vi "Simulation - Tank Level.vi"() -> ()   [LabVIEW 2023]
doc: "This example demonstrates a process simulation for a tank level. The process has added noise, valve deadband, lag, and deadtime. A level controller adjusts the inflow to a tank. An on/off valve serves as a drain that you can click on to operate. This s-valve represents a change in the process loading. You also can switch this VI from automatic control to manual control."
uses:
  <vilib>/addons/control/pid/pid.llb/PID Advanced (DBL).vi
  <vilib>/addons/control/pid/NI_PID_pid.lvlib
panel:
  in  "Tab Control":enum32{"Introduction", "Operation"}(tab)
  out "Flow sensor":bool
  in  "HV-101":bool
  out "tank level":dbl(slide) scale=0.0..100.0 scale format="%#.2g"
  out "Valve":bool
  in  "LCV-101":dbl(knob) scale=0.0..100.0
  in  "Auto":bool=TRUE
  out "Process Chart":T1(graph)={"initial PV"=18.934717983735947, "SP(%)"=34.59119496855346, "output"=100.0}
  in  "Setpoint":dbl(slide)=50.0 scale=0.0..100.0
  in  "PID parameters (LIC 101)":T2={"Kc"=10.0, "Ti (min)"=0.05, "Td (min)"=0.0} {"Td (min)" format="%#.6f"; "Ti (min)" format="%#.4f"; "Kc" format="%#.4f"}
  in  "Stop":bool
  # "Tank Level Control"
  # "Overview: This example demonstrates a process simulation for a tank level.  The process has added noise, valve deadband, lag, and deadtime.  A level controller adjusts the inflow to a tank.  An on/off valve serves as a drain that you can click on to operate.  This s-valve represents a change in the process loading.  You also can switch this VI from automatic control to manual control.\nInstructions:\n1. Run the VI.\n2. Verify the PID controller in closed-loop to track the setpoint.\n3. Change the setpoint to another value and verify the controller tracking the new setpoint.\n4. Apply a disturbance to the system by switching the valve HV 102 (click on the valve symbol). You will see the controller recovering fro the change.\n5. Change PID gains and see if you can improve its performance without going unstable.\n6. Switch to manual mode and see if you can control the level by changing the Valve LVC 101.\n7. Click Stop to stop the VI."
  # "ISA Symbology: The diagram uses the ISA Symbology used for control"
  # "Loop 101"
  # "Level Controller at the control room"
  # "Level Transmitter on the field"
  # "Level Control Valve on the field"
  # "Hand Control Valve on the field"
  # "HV"
  # "102"
  # "LCV"
  # "101"
  # "LIC"
  # "101"
  # "LT"
  # "101"
  # "Slow Leak"
  # "Click to operate"
  # "HV"
  # "102"
  # "LCV"
  # "101"
  # "LIC"
  # "101"
  # "LT"
  # "101"
  # "Manual"
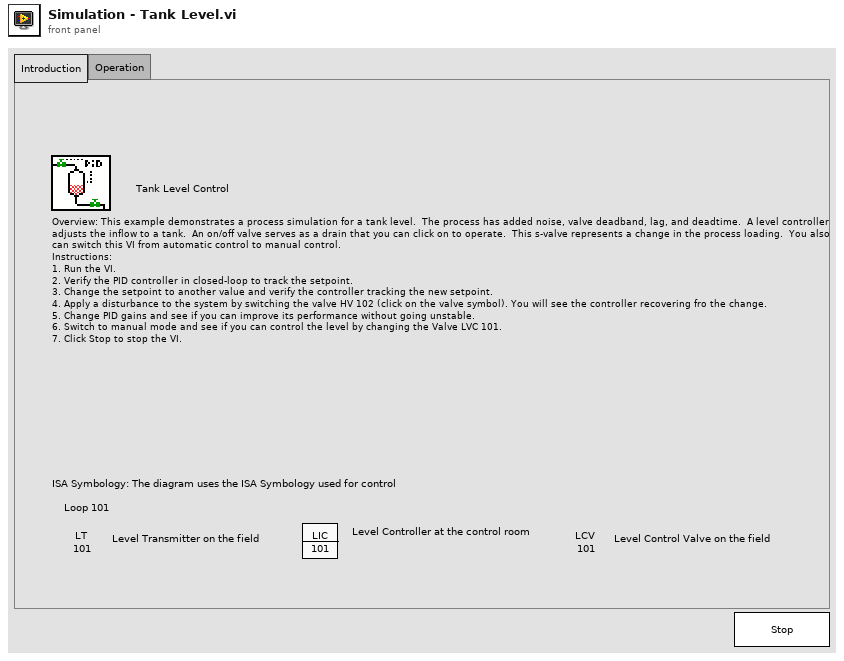
[diagram p1: front panel]
types:
  T1 = cluster{"initial PV":dbl, "SP(%)":dbl, "output":dbl}
  T2 = cluster{"Kc":dbl, "Ti (min)":dbl, "Td (min)":dbl}
  T3 = cluster{"static gain":dbl, "lag (s)":dbl, "deadtime (s)":dbl, "load":dbl, "deadband":dbl, "sensor noise":dbl, "initial PV":dbl, "plant noise":dbl}
  T4 = cluster{"Plant Output":dbl, "Setpoint":dbl, "output":dbl}
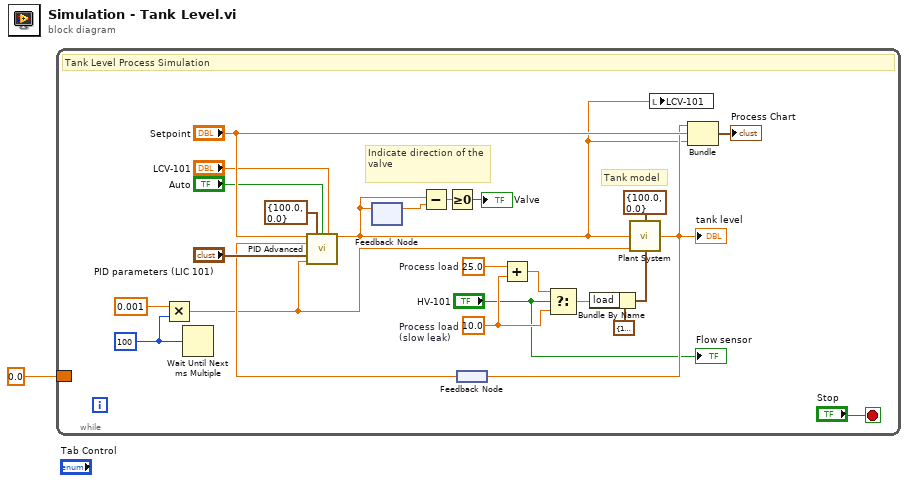
[diagram p0: block diagram]
diagram:
  n1 = while {
    border: 0.0 ("Plant Output") -> [_]
    stop <- "Stop" stop-if-true
    w12 = u32 100
    w4 = 25.0  # Process load
    w5 = 10.0  # Process load (slow leak)
    # "Tank model"
    # "Indicate direction of the valve"
    # "Tank Level Process Simulation"
    n2 = Multiply(x=0.001, y=w12) -> (x*y=w11:dbl)
    n3 = Wait Until Next ms Multiple(millisecond multiple=w12) -> ()  [unwired: 1 out]
    n4 = feedback #1() -> (w9:dbl)  [unwired: 1 in]
    n5 = feedback #2() -> (w14:dbl)
    n6 = call-poly <vilib>:"PID Advanced.vi"("setpoint"="Setpoint", "output range"=cluster{"output high":dbl, "output low":dbl} {"output high"=100.0, "output low"=0.0}, "auto? (T)"="Auto", "manual control"="LCV-101", "process variable"=w14, "PID gains"="PID parameters (LIC 101)", "dt (s)"=w11) -> ("output"=w8:dbl)  [unwired: 7 in, 1 out]
    n7 = feedback-in #1(w8) -> ()
    n8 = Subtract(x=w8, y=w9) -> (x-y=w7:dbl)
    n9 = Greater Or Equal To 0?(x=w7) -> (x >= 0?=→"Valve":bool)
    n10 = Add(x=w4, y=w5) -> (x+y=w3:dbl)
    n11 = Select(t=w3, s="HV-101", f=w5) -> (s? t:f=w16:dbl)
    n12 = Bundle By Name(cluster=T3 {"static gain"=1.5, "lag (s)"=18.0, "deadtime (s)"=1.0, "load"=0.0, "deadband"=1.0, "sensor noise"=0.0, "initial PV"=0.0, "plant noise"=5.0} ("process parameters"), "load"=w16) -> (w15:T3)
    n13 = call "Plant System.vi"("output saturation range"=cluster{"output high":dbl, "output low":dbl} {"output high"=100.0, "output low"=0.0}, "Plant Input"=w8, "dt (s)"=w11, "process parameters"=w15) -> ("Plant Output"=w10:dbl)  [unwired: 11 in]
    "tank level" <- w10
    n14 = feedback-in #2(w10) -> ()
    n15 = local write "LCV-101"(w8) -> ()
    n16 = Bundle("Plant Output"=w10, "Setpoint"="Setpoint", "output"=w8) -> (→"Process Chart":T4)  [unwired: 1 in]
    "Flow sensor" <- "HV-101"
  }
